vi "Parse Customer Name.vi"(10 "SR Cluster in":T1 {"Creation Date" format="%<%x>T"; "Last Updated" format="%<%x>T"}, 11 "HTML text in":string) -> (2 "SR Cluster out":T1 {"Creation Date" format="%<%x>T"; "Last Updated" format="%<%x>T"}, 3 "remaining string out":string)   [LabVIEW 2018]
uses:
  Type Defs/SR Cluster.ctl
  Type Defs/SR Status.ctl
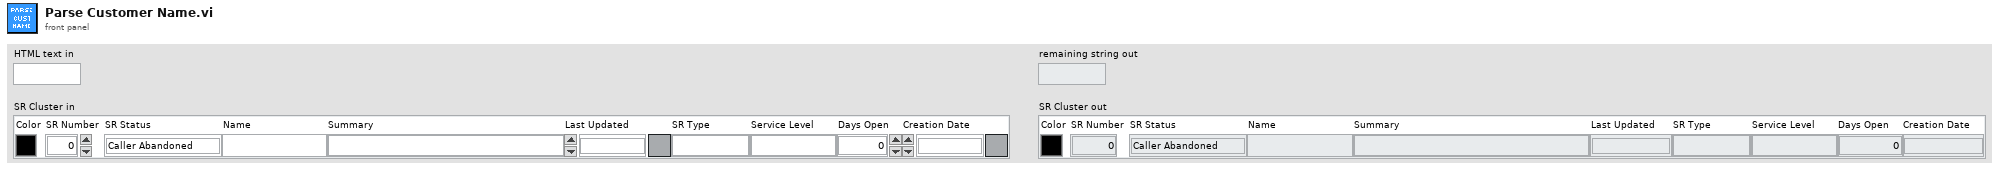
[diagram p1: front panel]
types:
  T1 = typedef "SR Cluster.ctl" = cluster{"Color":u32, "SR Number":i32, "SR Status":T2, "Name":string, "Summary":string, "Last Updated":timestamp, "SR Type":string, "Service Level":string, "Days Open":dbl, "Creation Date":timestamp}
  T2 = typedef "SR Status.ctl" = enum16{"Caller Abandoned", "Created in Error", "Expired", "Forum Resolved AE", "Forum Resolved Customer", "IN WORK", "IN WORK Collab with AES", "IN WORK Collab with PSE", "IN WORK Collab with SE", "IN WORK Customer Added Note", "IN WORK Escalation", "IN WORK Wait on Customer", "Open", "Potentially Resolved", "Presumed Resolved", "RMA Approved for Return", "Resolved", "Passed Off"}
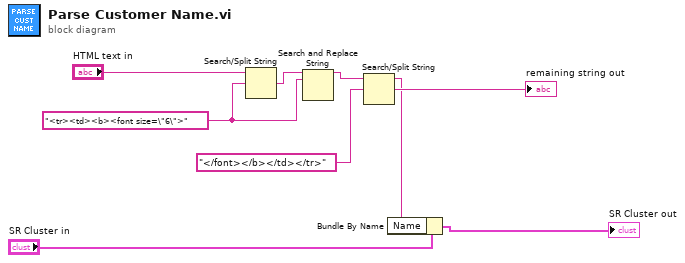
[diagram p0: block diagram]
diagram:
  w3 = "<tr><td><b><font size=\"6\">" ("search string/char (-)")
  n1 = Search/Split String(string="HTML text in", search string/char (-)=w3) -> (match + rest of string=w2:string)  [unwired: 1 in, 2 out]
  n2 = Search and Replace String(input string=w2, search string=w3) -> (result string=w4:string)  [unwired: 6 in, 3 out]
  n3 = Search/Split String(string=w4, search string/char (-)="</font></b></td></tr>") -> (substring before match=w8:string, match + rest of string=→"remaining string out":string)  [unwired: 1 in, 1 out]
  n4 = Bundle By Name(cluster="SR Cluster in", "Name"=w8) -> (→"SR Cluster out":T1)
